vi "Add.vi"(10 "y":dbl, 11 "x":dbl) -> (3 "X+Y":dbl)   [LabVIEW 2015, in "Math Library.lvlib"]
uses:
  Math Library.lvlib
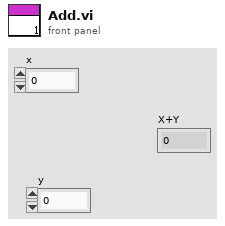
[diagram p1: front panel]
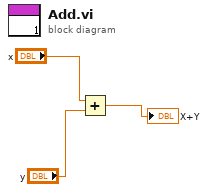
[diagram p0: block diagram]
diagram:
  n1 = Add(x="x", y="y") -> (x+y=→"X+Y":dbl)
